vi "GUID Lookup.vi"() -> ()   [LabVIEW 2015, in "Diagnostics Addon Shared.lvlib"]
doc: "Use this Global VI to access the GUIDs assigned to the page resources of the Custom Device."
uses:
  Diagnostics Addon Shared.lvlib
panel:
  in  "Tab Control":enum32{"GUIDs", "Constants", "Properties"}(tab)=enum."Constants"
  in  "DID Outputs GUID":string="a1b4f299-b02f-4aee-83c4-b2663edfc3d0"
  in  "DTC Control GUID":string="c7c1a7e9-77d4-474c-a0e9-38edab0be724"
  in  "Memory Location GUID":string="bcff0b3d-7243-4886-a340-96f6fb52a52d"
  in  "Memory Inputs GUID":string="09bcd3f1-7ebd-43d6-9f90-c7b275b290a5"
  in  "Memory Outputs GUID":string="8568ba9d-faad-4aba-a1fa-a7191ea76f8f"
  in  "Memory GUID":string="ddf9fde4-b7c4-46c2-b039-1cf8b908c912"
  in  "DID Inputs GUID":string="7aa10d41-82af-42f0-a422-22627e0c3946"
  in  "Diagnostics_Enable":string="4e42e445-e1c9-40fb-b144-894b15ca645a"
  in  "DTCs GUID":string="631db7b8-0b52-4af9-934d-144228c2dbd8"
  in  "PIDs GUID":string="1514cba4-fa1e-47dd-8223-616adb9fb21d"
  in  "Status GUID":string="f7446a49-c995-4f37-8203-8e2b918d40c6"
  in  "Commands GUID":string="14802196-9eef-416a-8ce6-e6467da1d504"
  in  "PID GUID":string="6b934904-49a9-4798-a421-a2da3be45ca1"
  in  "PID Inputs GUID":string="3a9eaf02-736d-4e36-bf88-b98c7e9eb737"
  in  "DPIDs GUID":string="186cc3e9-a602-40ff-b933-3b68f6fbfaf8"
  in  "DPID GUID":string="be84dd52-6fa5-4162-93da-bfddf126599b"
  in  "DTC GUID":string="7ba6be2c-4857-4b46-8446-f293283a3924"
  in  "Diagnostics_Disable":string="1dbbfb91-19dd-4678-8b23-0ef3a754a66d"
  in  "PID Outputs GUID":string="edf3a6ba-361e-4d29-8f85-616268b5a338"
  in  "IO GUID":string="340d50a8-4c77-4b9c-9e2b-69668480a08c"
  in  "Routine GUID":string="6fce7018-00fd-4fe4-bfd5-c0801fde7f06"
  in  "Signal GUID":string="813ed40a-6aa8-4ff9-92f7-887fb6dec76c"
  in  "Protected Signal GUID":string="edc2e041-ff43-4610-a968-1d89a067df1d"
  in  "DID GUID":string="465d9377-cb59-4ae9-97ed-bc842761823f"
  in  "Routine Start GUID":string="7299a859-e27a-4f6d-ab3a-db802fb4db39"
  in  "Routine Stop GUID":string="77ae2b93-bc49-4a11-9803-49f6a1a61766"
  in  "Routine Request GUID":string="ed43eaed-92e2-4ea6-9195-de19bee607ee"
  in  "IO Control GUID":string="0ac6196a-385b-4d7f-b227-6021e7d2e1e7"
  in  "Routines GUID":string="0ff37a6c-fd65-46dd-8b75-df84d7ab3dd8"
  in  "Response GUID":string="bc55b15e-e331-4782-b5d4-23fb44f573db"
  in  "Command GUID":string="37a28eab-899c-4060-83a1-bccb94c61935"
  in  "DIDs GUID":string="ae6faf55-1aff-4d2a-b6e8-d238aa342751"
  in  "Diagnostic Command Payload Bytes":string="Data Length"
  in  "Diagnostic Command Error Code":string="VeriStand Error"
  in  "Diagnostic Command Error Byte":string="Error Byte"
  in  "DTC Control Page":string="DTC Control"
  in  "Memory Page":string="Memory"
  in  "Response Page":string="Response"
  in  "Command Page":string="Command"
  in  "Routines Page":string="Routines"
  in  "Routine Start Page":string="Start"
  in  "Routine Stop Page":string="Stop"
  in  "Routine Request Page":string="Request"
  in  "CommandChannels":string[](array[string])=["Command", "MetaData1", "MetaData2", "MetaData3", "MetaData4"]
  in  "DTC_Signal Suffix":string[](array[string])=["_Timestamp", "_Value", "_Status", "_Failure"]
  in  "DIDs Page":string="DIDs"
  in  "DB Alias":string="Diagnostics_Addon_Temp_DB"
  in  "DTC_Signal Prefix":string="DTC_"
  in  "DTC_Signals to Create":i32=10
  in  "CD Version":string="5.0.0"
  in  "Inputs Page":string="Inputs"
  in  "DPIDs Page":string="DPIDs"
  in  "LookupTableSignalsPrefix":string="SignalDefs"
  in  "LookupTableConvertPrefix":string="Convert"
  in  "PIDs Page":string="PIDs"
  in  "DTCs Page":string="DTCs"
  in  "Status Page":string="Status"
  in  "Services Page":string="Services"
  in  "Commands Page":string="Commands"
  in  "DTCs_Masks":string="DTC Masks"
  in  "Data by Identifier Page":string="Data by Identifiers"
  in  "Diagnostic Command Success":string="Diagnostic Command Success"
  in  "CmdEngineSuffix":string="_BufferedCmds"
  in  "XNETEngineSuffix":string="_XNETEngine"
  in  "ResponseQKey":string="Response"
  in  "DTCs_# of DTCs":string="# of DTCs"
  in  "Outputs Page":string="Outputs"
  in  "IO Control Page":string="IO Control"
  in  "Type":string="Type"
  in  "CAN.Termination":string="Termination"
  in  "CAN.FillByte":string="FillByte"
  in  "CAN.FillFrame":string="FillFrame"
  in  "DTC.Order":string="ByteOrder"
  in  "DTC.AddByte":string="AddByte"
  in  "DTC.StatusByte":string="StatusByte"
  in  "DPID.PIDs":string="PIDs"
  in  "DPID.Speed":string="Speed"
  in  "Compiled.Settings":string="Compiled.Settings"
  in  "CAN.SecurityLevel":string="SecurityLevel"
  in  "CAN.SecurityDLL":string="SecurityDLL"
  in  "CAN.VWTPID":string="VWTPID"
  in  "CAN.Stream":string="Stream"
  in  "CAN.ReceiveUUDTID":string="ReceiveUUDTID"
  in  "CAN.ReceiveExt":string="ReceiveExt"
  in  "CAN.TransmitExt":string="TransmitExt"
  in  "CAN.ReceiveID":string="ReceiveID"
  in  "CAN.TransmitID":string="TransmitID"
  in  "CAN.Tranport":string="Tranport"
  in  "CAN.Protocol":string="Protocol"
  in  "CAN.BaudRate":string="BaudRate"
  in  "CAN.Interface":string="Interface"
  in  "Signal.Description":string="Description"
  in  "Signal.Units":string="Units"
  in  "Signal.Name":string="Name"
  in  "Signal.DefaultValue":string="DefaultValue"
  in  "Signal.ByteOrder":string="ByteOrder"
  in  "Signal.DataType":string="DataType"
  in  "Signal.Max":string="Max"
  in  "Signal.Min":string="Min"
  in  "Signal.ScalingOffset":string="ScalingOffest"
  in  "Signal.ScalingFactor":string="ScalingFactor"
  in  "Signal.Length":string="Length"
  in  "Enable 986x":string="Enable 986x"
  in  "RIO Device 986x":string="RIO Device 986x"
  in  "RT Bitfile Location":path=path "c:/ni-rt/NIVeriStand/XNET"
  in  "Bitfile 986x":string="Bitfile 986x"
  in  "DTC.DTCByte":string="DTCByte"
  in  "ID":string="ID"
  in  "Signal.StartBit":string="StartBit"
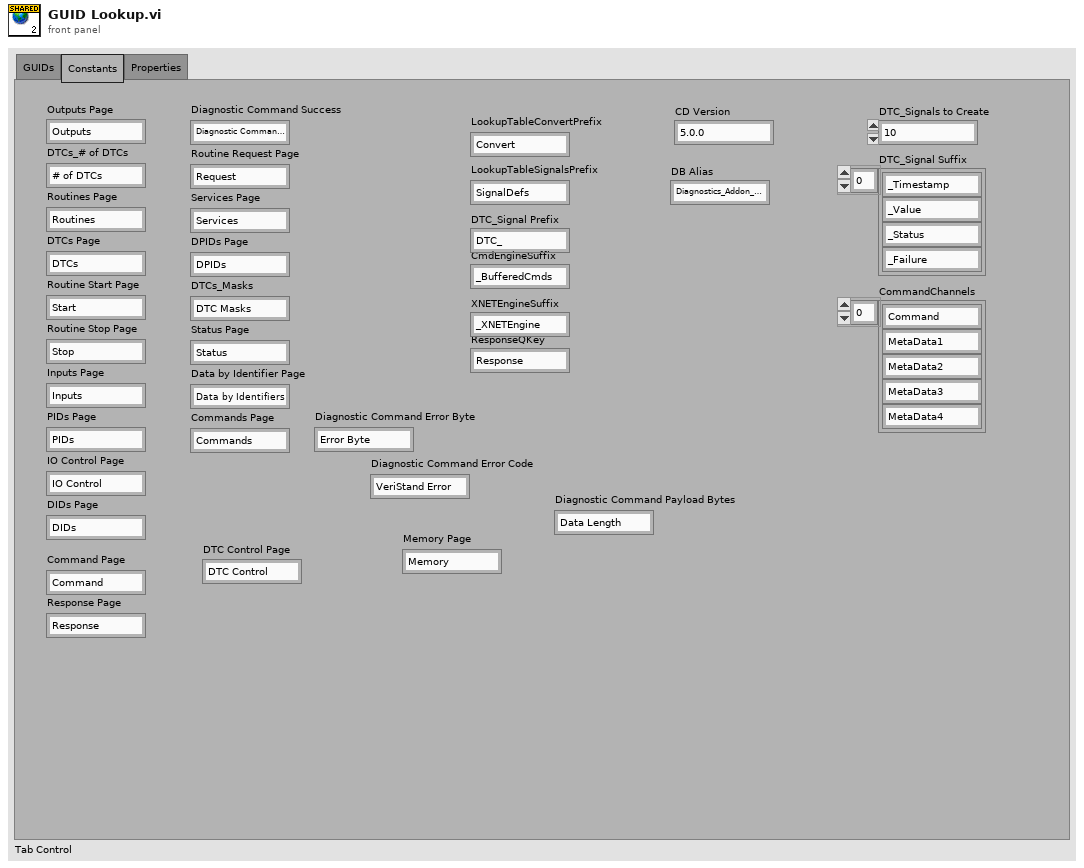
[diagram p1: front panel]
diagram:
